vi "Boolean to Matlab String.vi"(8 "error in (no error)":errorcluster, 10 "Data":bool, 11 "Variable name":string) -> (0 "error out":errorcluster, 3 "String":string)   [LabVIEW 2011, in "Matlab API.lvlib"]
uses:
  Matlab API.lvlib
panel:
  out "Array":u8[](array[numeric]) format="%x"
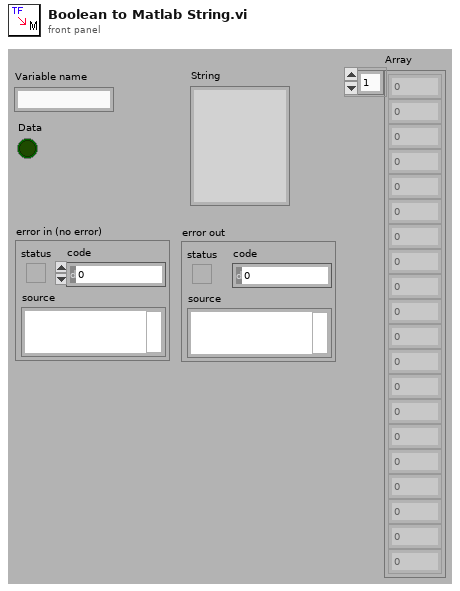
[diagram p1: front panel]
types:
  T1 = enum16{"big-endian, network order", "native, host order", "little-endian"}
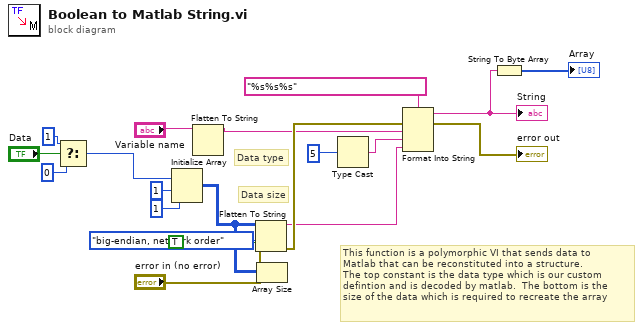
[diagram p0: block diagram]
diagram:
  # "Data size"
  # "Data type"
  # "This function is a polymorphic VI that sends data to\nMatlab that can be reconstituted into a structure.\nThe top constant is the data type which is our custom\ndefintion and is decoded by matlab.  The bottom is the\nsize of the data which is required to recreate the array"
  n1 = Select(t=u8 1, s="Data", f=u8 0) -> (s? t:f=w3:u8)
  n2 = Initialize Array(w3, 1 ("dimension size"), 1 ("dimension size")) -> (w5:u8[][])
  n3 = Flatten To String(anything="Variable name") -> (data string=w11:string)  [unwired: 1 in, 4 out]
  n4 = Flatten To String(anything=w5, prepend array or string size? (T)=TRUE, byte order (0:big-endian, network order)=T1."big-endian, network order", error in (no error)="error in (no error)") -> (data string=w8:string, error out=w17:errorcluster)  [unwired: 1 out]
  n5 = Array Size(array=w5) -> ()  [unwired: 1 out]
  n6 = Type Cast(x=5 ("input 2")) -> (*(type *) &x=w13:string)  [unwired: 1 out]
  n7 = Format Into String(format string="%s%s%s", error in=w17, w11, w13, w8) -> (resulting string=w14:string, error out=→"error out":errorcluster)  [unwired: 1 in]
  "String" <- w14
  n8 = String To Byte Array(string=w14) -> (unsigned byte array=→"Array":u8[])
